vi "Config Root.vi"(8 "error in (no error)":errorcluster, 11 "App in":refnum<class "App.lvclass">) -> (0 "error out":errorcluster, 1 "Main Filename":string, 2 "Config Root":path, 3 "App out":refnum<class "App.lvclass">)   [LabVIEW 2020, in "Volatus.lvlib" / "App.lvclass"]
uses:
  App.lvclass
  App.lvclass/App.ctl
  <vilib>/Utility/config.llb/NI_LVConfig.lvlib
  <vilib>/Utility/config.llb/Read Key (String).vi
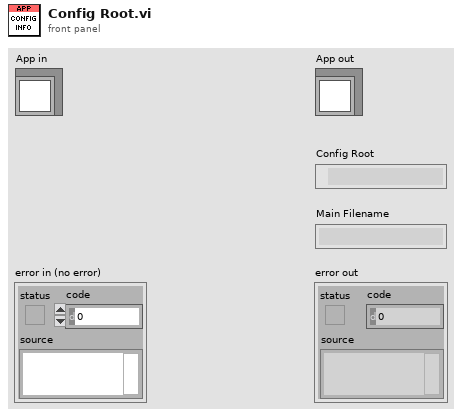
[diagram p1: front panel]
types:
  T1 = typedef "NI_LVConfig.lvlib/Config Data RefNum.ctl" = refnum<k1>
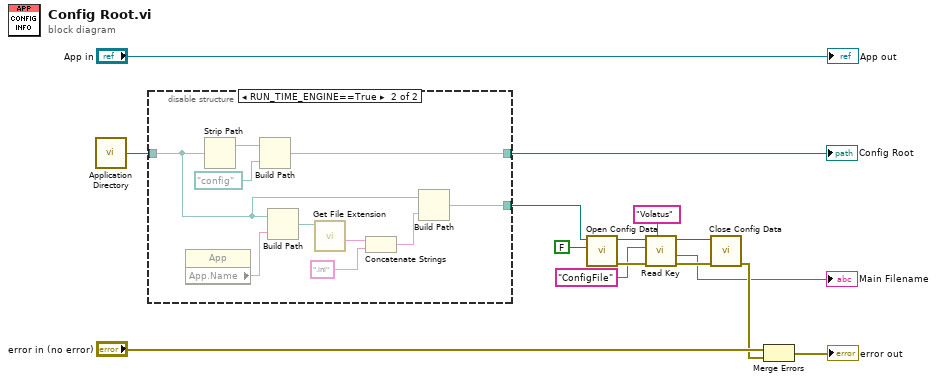
[diagram p0: block diagram]
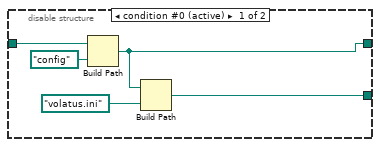
[diagram p2: hidden frame]
diagram:
  n1 = call <vilib>:"Application Directory.vi"() -> ("Application Directory"=w13:path)
  n2 = disable-structure shown="RUN_TIME_ENGINE==True" {
    disable-tunnel: w13 -> [w20 w22]
    disable-tunnel: [w18 w28] -> w12
    disable-tunnel: [w16 w21] -> w3
    frame condition #0 (active) {
      n3 = Build Path(base path=w20, name or relative path=path "config") -> (appended path=w18:path)
      n4 = Build Path(base path=w18, name or relative path=path "volatus.ini") -> (appended path=w16:path)
    }
    frame condition #1 {
      n5 = property class="App"() -> ("App.Name"=w27:string)  [unwired: 2 in, 2 out]
      n6 = Strip Path(path=w22) -> (stripped path=w30:path)  [unwired: 1 out]
      n7 = Build Path(base path=w30, name or relative path=path "config") -> (appended path=w28:path)
      n8 = Build Path(base path=w22, name or relative path=w27) -> (appended path=w26:path)
      n9 = call <vilib>:"Get File Extension.vi"("file"=w26) -> ("filename without extension"=w25:string)  [unwired: 6 in, 4 out]
      n10 = Concatenate Strings(w25, ".ini") -> (w23:string)
      n11 = Build Path(base path=w22, name or relative path=w23) -> (appended path=w21:path)
    }
  }
  "Config Root" <- w12
  n12 = call <vilib>:"Open Config Data.vi"("create file if necessary (T)"=FALSE, "configuration file path"=w3) -> ("error out"=w8:errorcluster, "refnum"=w9:T1)  [unwired: 7 in, 1 out]
  n13 = call-poly <vilib>:"Read Key.vi"("section"="Volatus", "error in (no error)"=w8, "key"="ConfigFile", "refnum"=w9) -> ("error out"=w7:errorcluster, "value"=→"Main Filename":string, "refnum out"=w10:T1)  [unwired: 4 in, 1 out]
  n14 = call <vilib>:"Close Config Data.vi"("error in (no error)"=w7, "refnum"=w10) -> ("error out"=w2:errorcluster)  [unwired: 8 in, 1 out]
  n15 = Merge Errors("error in (no error)", w2) -> (→"error out":errorcluster)
  "App out" <- "App in"
